vi "PH_Beckhoff-16BB_Testtool.ProcCases.vi"(0 "i ref in":refnum<vi>, 1 "selector":string, 2 "Data":T1, 3 "call cluster":T2={"Object"="", "Selector"="", "CallType"=enum."synchronous", "Async Object"="", "Async Selector"="", "Data Descriptor"="", "Data"=[], "Error #"=0, "Expire"=0}, 5 "error in (no error)":errorcluster) -> (14 "i ref out":refnum<vi>, 17 "answer cluster":T2={"Object"="", "Selector"="", "CallType"=enum."synchronous", "Async Object"="", "Async Selector"="", "Data Descriptor"="", "Data"=[], "Error #"=0, "Expire"=0}, 19 "error out":errorcluster)   [LabVIEW 2014, in "PH_Beckhoff-16BB_Testtool.lvlib"]
doc: "This method is called by a process from within the default case in the event loop. The methods of a class that are linked to events will be called from THIS method. Add your code here."
uses:
  PH_Beckhoff-16BB_Testtool.lvlib
  CS_Core/CSSystem/CoreDefs/CoreDefs.call_type.ctl
  CS_Core/BaseProcess/BaseProcess.descriptor string definition.ctl
  CS_Core/CSSystem/CoreDefs/CoreDefs.rawDataType.ctl
  CS_Core/CSSystem/CoreLib/CoreLib.string 2 byte array.vi
  CS_Core/BaseProcess/BaseProcess.lvlib
  PH_Basics/PH_Common/PH_Common.lvlib
  CS_Core/CAEObj/CAEObj.lvlib
  CS_Core/CSSystem/CoreLib/CoreLib.lvlib
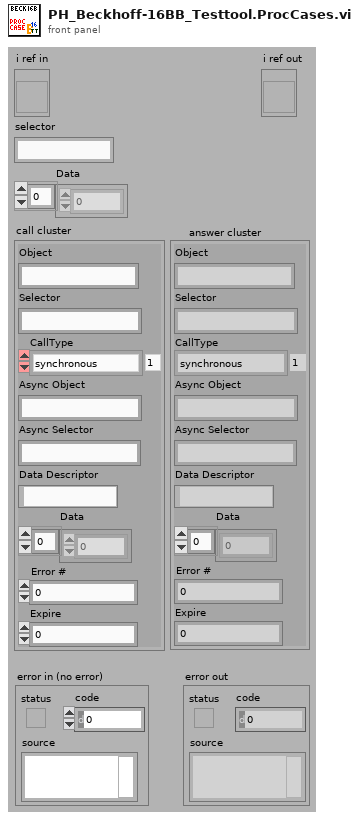
[diagram p1: front panel]
types:
  T1 = typedef "CoreDefs.rawDataType.ctl" = i8[]
  T2 = typedef "CoreDefs.call_type.ctl" = cluster{"Object":string, "Selector":string, "CallType":enum16{"simple", "synchronous", "asynchronous"}, "Async Object":string, "Async Selector":string, "Data Descriptor":T3, "Data":T1, "Error #":i32, "Expire":u32}
  T3 = typedef "BaseProcess.lvlib/BaseProcess.descriptor string definition.ctl" = string
  T4 = typedef "PH_Beckhoff-16BB_Testtool.lvlib/PH_Beckhoff-16BB_Testtool.i attribute.ctl" = cluster{"GUI Refs":refnum<vi>[], "16BB Instance":string}
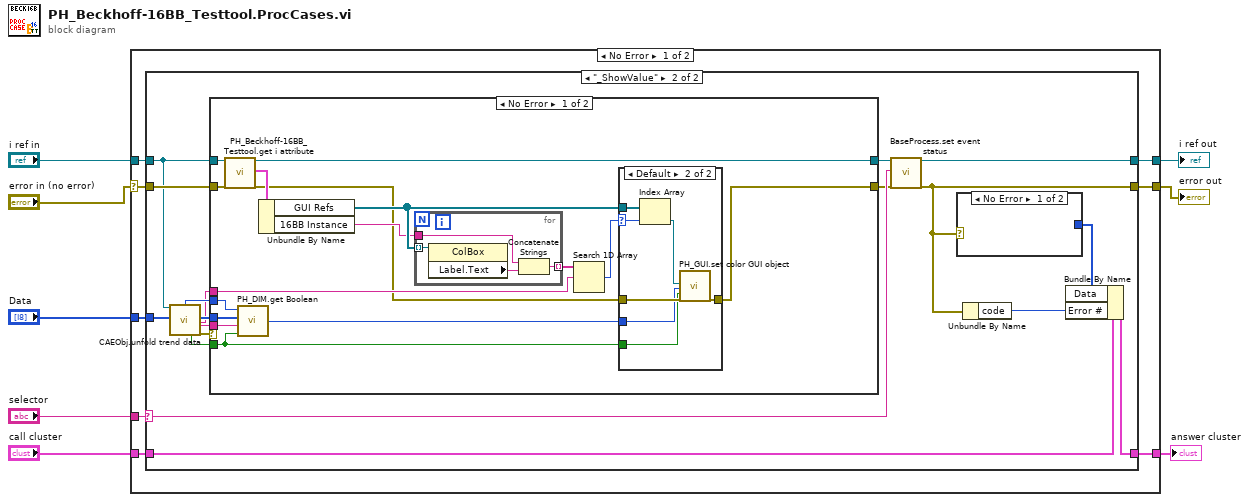
[diagram p0: block diagram]
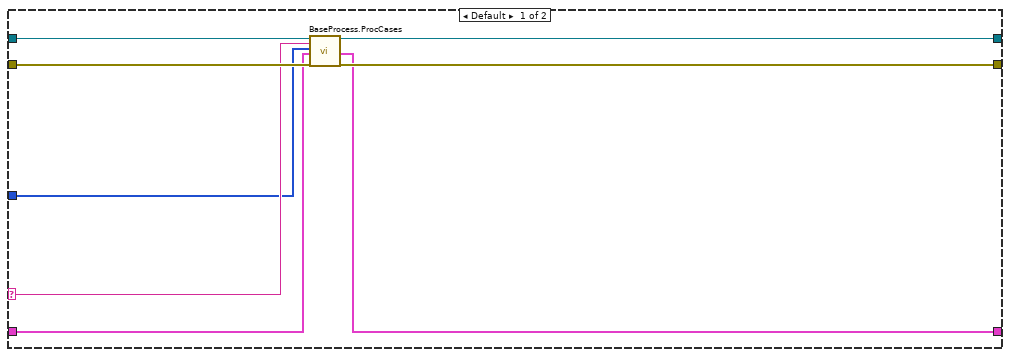
[diagram p2: hidden frame]
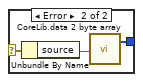
[diagram p3: hidden frame]
diagram:
  n1 = case shown="No Error" "error in (no error)" {
    selector: "error in (no error)" -> [w9 w77]
    tunnel: "selector" -> [w16 _]
    tunnel: [w15 w76] -> w7
    tunnel: "call cluster" -> [w14 w76]
    tunnel: "i ref in" -> [w13 w78]
    tunnel: [w12 w78] -> w4
    tunnel: [w11 w77] -> w3
    tunnel: "Data" -> [w10 _]
    frame No Error {
      n2 = case shown="\"_ShowValue\"" w16 {
        selector: w16 -> [w19 w32]
        tunnel: w10 -> [w17 w41]
        tunnel: w13 -> [w18 w40]
        tunnel: [w24 w29] -> w12
        tunnel: w14 -> [w20 w28]
        tunnel: [w21 w27] -> w15
        tunnel: w9 -> [w23 w42]
        tunnel: [w22 w26] -> w11
        frame Default {
          n3 = call "BaseProcess.ProcCases.vi"("i ref in"=w18, "selector"=w19, "Data"=w17, "call cluster"=w20, "error in (no error)"=w23) -> ("i ref out"=w24:refnum<vi>, "answer cluster"=w21:T2, "error out"=w22:errorcluster)  [unwired: 12 in]
        }
        frame "_ShowValue" {
          n4 = call "CAEObj.unfold trend data.vi"("i ref in"=w40, "raw trend data"=w41) -> ("quality"=w35:i32, "no link"=w36:bool, "data"=w38:i8[], "serviceName"=w25:string, "typeDescriptor"=w37:string, "error out"=w39:errorcluster)  [unwired: 9 in, 3 out]
          n5 = case shown="No Error" w39 {
            tunnel: [w47 w75] -> w31
            tunnel: w40 -> [w61 w75]
            tunnel: w42 -> [w60 w74]
            tunnel: [w53 w74] -> w30
            tunnel: w38 -> [w57 _]
            tunnel: w37 -> [w56 _]
            tunnel: w36 -> [w54 _]
            tunnel: w35 -> [w55 _]
            tunnel: w25 -> [w50 _]
            frame No Error {
              n6 = call "PH_Beckhoff-16BB_Testtool.get i attribute.vi"("i ref in"=w61, "error in (no error)"=w60) -> ("i ref out"=w47:refnum<vi>, "i attribute"=w59:T4, "error out"=w46:errorcluster)  [unwired: 15 in]
              n7 = call "PH_DIM.get Boolean.vi"("no link"=w54, "typeDescriptor"=w56, "data"=w57, "quality"=w55) -> ("Value"=w58:i32)
              n8 = Unbundle By Name(w59) -> ("GUI Refs"=w52:refnum<vi>[], "16BB Instance"=w48:string)
              n9 = for {
                tunnel: w52 -> [w73] mode=indexing
                tunnel: w48 -> [w72]
                tunnel: [w70] -> w51 mode=indexing
                n10 = property class="ColBox"(reference=w73) -> ("Label.Text"=w71:string)  [unwired: 1 in, 2 out]
                n11 = Concatenate Strings(w72, w71) -> (w70:string)
              }
              n12 = Search 1D Array(1D array=w51, element=w50) -> (index of element=w49:i32)  [unwired: 1 in]
              n13 = case shown="Default" w49 {
                selector: w49 -> [_ w63]
                tunnel: w46 -> [w62 w69]
                tunnel: w58 -> [_ w68]
                tunnel: w54 -> [_ w67]
                tunnel: [w62 w66] -> w53
                tunnel: w52 -> [_ w65]
                frame -1 {
                }
                frame Default {
                  n14 = Index Array(array=w65, index=w63) -> (element=w64:refnum<vi>)
                  n15 = call "PH_GUI.set color GUI object.vi"("GUI object Ref"=w64, "State"=w68, "Blinking? (false)"=w67, "error in (no error)"=w69) -> ("error out"=w66:errorcluster)  [unwired: 15 in]
                }
              }
            }
            frame Error {
            }
          }
          n16 = call "BaseProcess.set event status.vi"("i ref in"=w31, "EventStatus"=w32, "error in (no error)"=w30) -> ("i ref out"=w29:refnum<vi>, "error out"=w26:errorcluster)  [unwired: 14 in, 1 out]
          n17 = case shown="No Error" w26 {
            selector: w26 -> [_ w45]
            tunnel: [_ w43] -> w33
            frame No Error {
            }
            frame Error {
              n18 = Unbundle By Name(w45) -> ("source"=w44:string)
              n19 = call-poly "CoreLib.data 2 byte array.vi"("string"=w44) -> ("byteArray out"=w43:T1)  [unwired: 18 in]
            }
          }
          n20 = Unbundle By Name(w26) -> ("code"=w34:i32)
          n21 = Bundle By Name(cluster=w28, "Data"=w33, "Error #"=w34) -> (w27:T2)
        }
      }
    }
    frame Error {
    }
  }
  "answer cluster" <- w7
  "i ref out" <- w4
  "error out" <- w3
